vi "Window.vi"() -> ()   [LabVIEW 2014]
uses:
  <vilib>/ErrorRing/Error Ring.xnode
  <vilib>/Utility/error.llb/Error Cluster From Error Code.vi
  AnalysisPluginsBase.lvclass
  Typedefs/clSampleData.ctl
panel:
  out "error out":errorcluster
  in  "error in (no error)":errorcluster
  out "Analysis Out":refnum<class "AnalysisPluginsBase.lvclass">
  in  "Analysis In":refnum<class "AnalysisPluginsBase.lvclass">
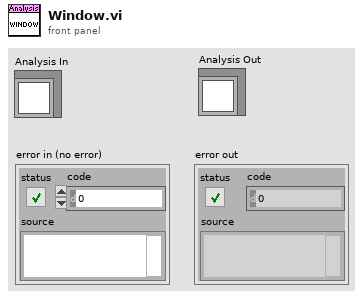
[diagram p1: front panel]
types:
  T1 = typedef "AnalysisPlugins.lvlib/AnalysisPluginsBase.lvclass/clSampleData.ctl" = cluster{"Timestamp":ext, "SampleDataInput":cluster{"dSampleData":dbl[], "iActualPts":i32}[]}
  T2 = typedef "AnalysisPlugins.lvlib/AnalysisPluginsBase.lvclass/clConfig.ctl" = cluster{"F0":u32, "SettlingTime":dbl, "AnalysisCycles":dbl, "SampleRate":dbl, "NumChannels":u32, "TsOffset":enum16{"start", "middle", "end"}}
  T3 = typedef "clWindowData.ctl" = cluster{"Timestamp":ext, "Samples":dbl[][], "Window Valid":bool}
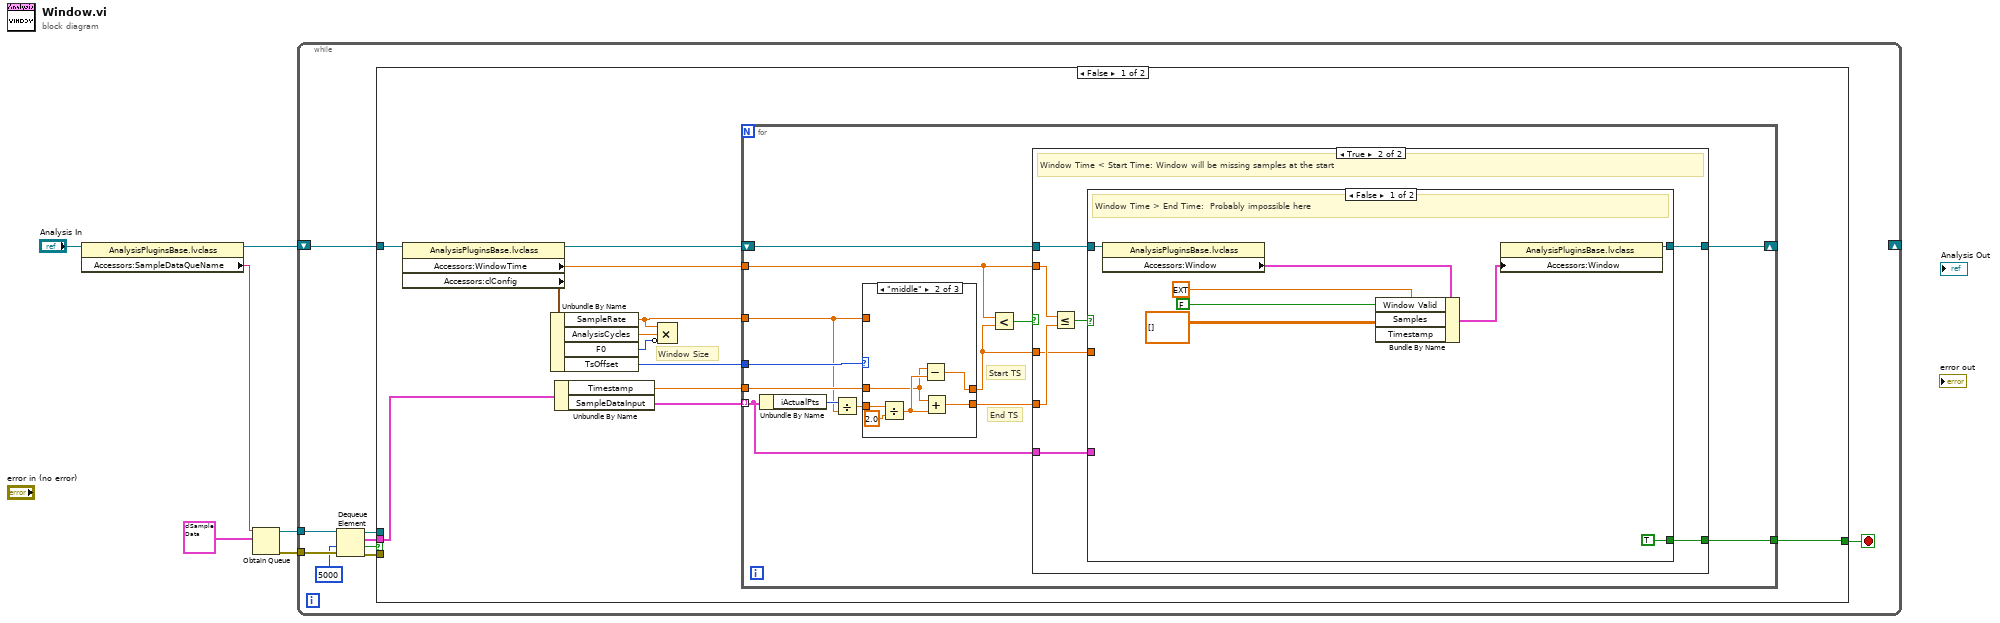
[diagram p0: block diagram]
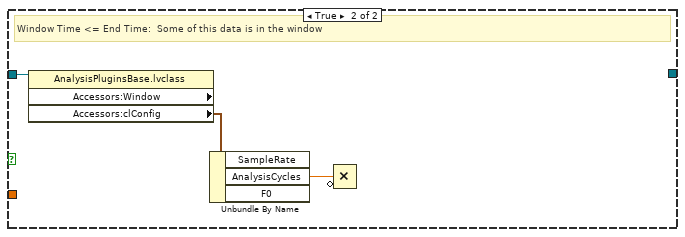
[diagram p3: hidden frame]
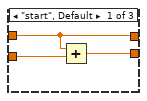
[diagram p4: hidden frame]
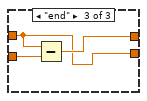
[diagram p5: hidden frame]
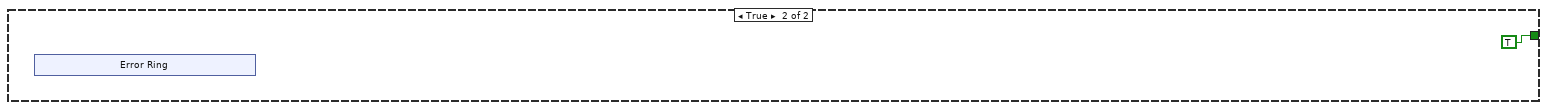
[diagram p6: hidden frame]
diagram:
  n1 = property class="AnalysisPluginsBase.lvclass"(reference="Analysis In") -> (reference out=w4:refnum<class "AnalysisPluginsBase.lvclass">, "Accessors:SampleDataQueName"=w5:string)  [unwired: 1 in, 1 out]
  n2 = Obtain Queue(name (unnamed)=w5, element data type=T1 {"Timestamp"=0.0, "SampleDataInput"=[]} ("clSampleData")) -> (queue out=w3:refnum<queue>, error out=w2:errorcluster)  [unwired: 3 in, 1 out]
  n3 = while {
    shift-right: _ -> [_]
    shift-left: w4 -> [w8]
    tunnel: w3 -> [w15]
    tunnel: w2 -> [w14]
    stop <- w7 stop-if-true
    n4 = Dequeue Element(queue=w15, timeout in ms (-1)=5000, error in (no error)=w14) -> (queue out=w10:refnum<queue>, element=w9:T1, timed out?=w12:bool, error out=w11:errorcluster)
    n5 = case shown="False" w12 {
      tunnel: w11 -> [_ _]
      tunnel: w10 -> [_ _]
      tunnel: w9 -> [w26 _]
      tunnel: w8 -> [w27 _]
      tunnel: [w16 TRUE] -> w7
      frame False {
        # "Window Size"
        n6 = property class="AnalysisPluginsBase.lvclass"(reference=w27) -> (reference out=w17:refnum<class "AnalysisPluginsBase.lvclass">, "Accessors:WindowTime"=w18:dbl, "Accessors:clConfig"=w25:T2)  [unwired: 1 in, 1 out]
        n7 = Unbundle By Name(w25) -> ("SampleRate"=w19:dbl, "AnalysisCycles"=w24:dbl, "F0"=w23:u32, "TsOffset"=w21:enum16{"start", "middle", "end"})
        n8 = Unbundle By Name(w26) -> ("Timestamp"=w20:ext, "SampleDataInput"=w22:cluster{"dSampleData":dbl[], "iActualPts":i32}[])
        n9 = Compound Arithmetic op=MULTIPLY(w19, w24, invert w23) -> ()  [unwired: 1 out]
        n10 = for {
          tunnel: w22 -> [w29] mode=indexing
          tunnel: w21 -> [w40]
          tunnel: w20 -> [w39]
          tunnel: w19 -> [w37]
          tunnel: w18 -> [w32]
          shift-right: [w30] -> _
          shift-left: w17 -> [w34]
          tunnel: [w31] -> w16
          # "Start TS"
          # "End TS"
          n11 = Unbundle By Name(w29) -> ("iActualPts"=w38:i32)
          n12 = Divide(x=w38, y=w37) -> (x/y=w36:dbl)
          n13 = case shown="\"middle\"" w40 {
            tunnel: w39 -> [w61 w65 w69]
            tunnel: w37 -> [_ _ _]
            tunnel: [w62 w63 w69] -> w33
            tunnel: [w61 w64 w70] -> w28
            tunnel: w36 -> [w60 w68 w71]
            frame "start", Default {
              n14 = Add(x=w61, y=w60) -> (x+y=w62:ext)
            }
            frame "middle" {
              n15 = Divide(x=w68, y=2.0) -> (x/y=w66:dbl)
              n16 = Subtract(x=w65, y=w66) -> (x-y=w64:ext)
              n17 = Add(x=w65, y=w66) -> (x+y=w63:ext)
            }
            frame "end" {
              n18 = Subtract(x=w69, y=w71) -> (x-y=w70:ext)
            }
          }
          n19 = Less?(x=w32, y=w28) -> (x < y?=w35:bool)
          n20 = case shown="True" w35 {
            tunnel: w34 -> [_ w45]
            tunnel: w33 -> [_ w47]
            tunnel: w32 -> [_ w48]
            tunnel: [_ w44] -> w31
            tunnel: [_ w43] -> w30
            tunnel: w29 -> [_ w42]
            tunnel: w28 -> [_ w41]
            frame False {
            }
            frame True {
              # "Window Time < Start Time: Window will be missing samples at the start"
              n21 = Less Or Equal?(x=w48, y=w47) -> (x <= y?=w46:bool)
              n22 = case shown="False" w46 {
                tunnel: w45 -> [w52 w59]
                tunnel: [TRUE _] -> w44
                tunnel: [w49 _] -> w43
                tunnel: w42 -> [_ _]
                tunnel: w41 -> [_ _]
                frame False {
                  # "Window Time > End Time:  Probably impossible here"
                  n23 = property class="AnalysisPluginsBase.lvclass"(reference=w52) -> ("Accessors:Window"=w51:T3)  [unwired: 1 in, 2 out]
                  n24 = Bundle By Name(cluster=w51, "Window Valid"=FALSE, "Samples"=dbl[][] [], "Timestamp"=ext 0.0) -> (w50:T3)
                  n25 = property class="AnalysisPluginsBase.lvclass"("Accessors:Window"=w50) -> (reference out=w49:refnum<class "AnalysisPluginsBase.lvclass">)  [unwired: 2 in, 1 out]
                }
                frame True {
                  # "Window Time <= End Time:  Some of this data is in the window"
                  n26 = property class="AnalysisPluginsBase.lvclass" props=["Accessors:Window", "Accessors:clConfig"](reference=w59) -> ("Accessors:clConfig"=w58:T2)  [unwired: 1 in, 3 out]
                  n27 = Unbundle By Name(w58) -> ("AnalysisCycles"=w57:dbl)  [unwired: 2 out]
                  n28 = Compound Arithmetic op=MULTIPLY(w57) -> ()  [unwired: 2 in, 1 out]
                }
              }
            }
          }
        }
      }
      frame True {
        n29 = xnode "Error Ring"() -> ()  [unwired: 1 out]
      }
    }
  }
